vi "PH_AxisGUI_BaseClass.Set Setting depending Captions.vi"(0 "i ref out":refnum<vi>, 5 "error in":errorcluster) -> (14 "i ref out":refnum<vi>, 19 "error out":errorcluster)   [LabVIEW 2014, in "PH_AxisGUI_BaseClass.lvlib"]
doc: "This VI acts on GUI elements."
uses:
  PH_AxisGUI_BaseClass.lvlib
  PH_Common/PH_Common.lvlib
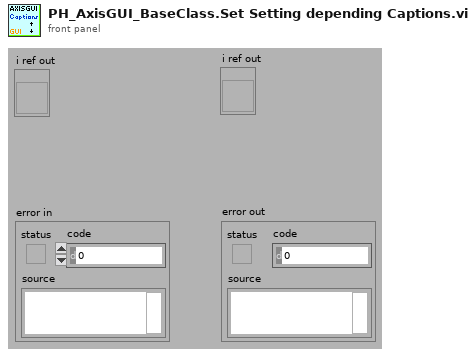
[diagram p1: front panel]
types:
  T1 = typedef "PH_AxisGUI_BaseClass.lvlib/PH_AxisGUI_BaseClass.i attribute.ctl" = cluster{"Axes":T2[]}
  T2 = typedef "PH_AxisGUI_BaseClass.lvlib/PH_AxisGUI_BaseClass.Axis Attributes.ctl" = cluster{"Axis GUI Refs":T3, "Address":T4, "Name":string, "Label \"Back\"":string, "Labell \"Forth\"":string, "Moving?":bool}
  T3 = typedef "PH_AxisGUI_BaseClass.lvlib/PH_AxisGUI_BaseClass.Axis GUI Refs.ctl" = cluster{"Back":refnum<vi>, "Forth":refnum<vi>, "Status":refnum<vi>, "Target":refnum<vi>, "Address":refnum<vi>, "Status Bar":refnum<vi>, "Settings":refnum<vi>, "Activity":refnum<vi>, "Clear Error":refnum<vi>}
  T4 = typedef "PH_Stepmotor_BaseClass.lvlib/PH_Stepmotor_BaseClass.Axis Address.ctl" = cluster{"Instance":string, "Motor Nr":i32}
  T5 = typedef "PH_Stepmotor_BaseClass.lvlib/PH_Stepmotor_BaseClass.Axis Settings.ctl" = cluster{"Sign change":bool, "Width":dbl, "Calibration":dbl, "Unit":string, "Motor Type":T6, "Unit Width":string, "Unit CF":string}
  T6 = typedef "PH_Stepmotor_BaseClass.lvlib/PH_Stepmotor_BaseClass.Motor Type.ctl" = enum16{"Unspecific", "OWIS 49.120.2633", "OWIS 49.060.1033", "OWIS 43.040.2558", "Diamond Motion 2200 series", "OWIS 49.120.266B.MV6", "Calorimeter", "Linear Stage 1", "MICOS VT-80", "MICOS VT-80 S", "Standa Rotstage nt0.95A", "PUF RA 320.200", "PUF RA 800.200", "PUF RA 800.400", "PUF RA 400.50", "1324.nn.800.50", "1324.n9c.800.50", "1324.nn.320.200", "1324.nn.400.200", "1324.nn.800.200", "1324.nn.400.50", "1324.8c9c.800.50", "1324.8c9c.400.200"}
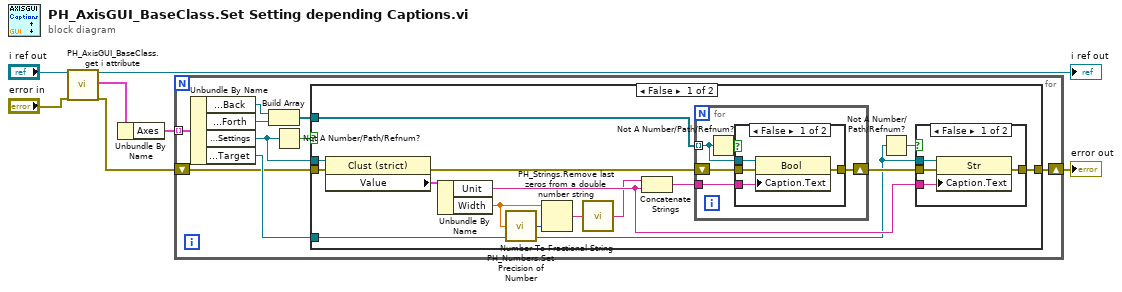
[diagram p0: block diagram]
diagram:
  n1 = call "PH_AxisGUI_BaseClass.get i attribute.vi"("i ref in"="i ref out", "error in (no error)"="error in") -> ("i ref out"=→"i ref out":refnum<vi>, "i attribute"=w2:T1, "error out"=w4:errorcluster)  [unwired: 15 in]
  n2 = Unbundle By Name(w2) -> ("Axes"=w1:T2[])
  n3 = for {
    shift-right: [w14] -> w3
    shift-left: w4 -> [w10]
    tunnel: w1 -> [w13] mode=indexing
    n4 = Unbundle By Name(w13) -> ("Axis GUI Refs.Back"=w16:refnum<vi>, "Axis GUI Refs.Forth"=w15:refnum<vi>, "Axis GUI Refs.Settings"=w8:refnum<vi>, "Axis GUI Refs.Target"=w12:refnum<vi>)
    n5 = Build Array(w16, w15) -> (w11:refnum<vi>[])
    n6 = Not A Number/Path/Refnum?(number/path/refnum=w8) -> (NaN/Path/Refnum?=w9:bool)
    n7 = case shown="False" w9 {
      tunnel: [w26 w47] -> w14
      tunnel: w12 -> [w25 _]
      tunnel: w8 -> [w24 _]
      tunnel: w11 -> [w23 _]
      tunnel: w10 -> [w22 w47]
      frame False {
        n8 = property class="Clust (strict)"(reference=w24, error in=w22) -> (error out=w21:errorcluster, "Value"=w31:T5)  [unwired: 1 out]
        n9 = Unbundle By Name(w31) -> ("Unit"=w28:string, "Width"=w18:dbl)
        n10 = call "PH_Numbers.Set Precision of Number.vi"("Number"=w18) -> ("Precision"=w17:i16)
        n11 = Number To Fractional String(number=w18, precision (6)=w17) -> (F-format string=w20:string)  [unwired: 2 in]
        n12 = call "PH_Strings.Remove last zeros from a double number string.vi"("String in"=w20) -> ("String out"=w19:string)
        n13 = Concatenate Strings(w19, w28) -> (w30:string)
        n14 = for {
          tunnel: w23 -> [w38] mode=indexing
          tunnel: w30 -> [w37]
          shift-right: [w40] -> w27
          shift-left: w21 -> [w41]
          n15 = Not A Number/Path/Refnum?(number/path/refnum=w38) -> (NaN/Path/Refnum?=w39:bool)
          n16 = case shown="False" w39 {
            tunnel: w41 -> [w45 w46]
            tunnel: [w44 w46] -> w40
            tunnel: w38 -> [w43 _]
            tunnel: w37 -> [w42 _]
            frame False {
              n17 = property class="Bool"(reference=w43, error in=w45, "Caption.Text"=w42) -> (error out=w44:errorcluster)  [unwired: 1 out]
            }
            frame True {
            }
          }
        }
        n18 = Not A Number/Path/Refnum?(number/path/refnum=w25) -> (NaN/Path/Refnum?=w29:bool)
        n19 = case shown="False" w29 {
          tunnel: w27 -> [w35 w36]
          tunnel: [w34 w36] -> w26
          tunnel: w25 -> [w33 _]
          tunnel: w28 -> [w32 _]
          frame False {
            n20 = property class="Str"(reference=w33, error in=w35, "Caption.Text"=w32) -> (error out=w34:errorcluster)  [unwired: 1 out]
          }
          frame True {
          }
        }
      }
      frame True {
      }
    }
  }
  "error out" <- w3
